vi "左相机穿管检测CCD1.vi"(8 "error in (no error)":errorcluster caption="错误输入（无错误）", 11 "名称或相对路径":string="Template Program") -> (0 "error in (no error) 2":errorcluster caption="错误输入（无错误）")   [LabVIEW 2017]
uses:
  Picture/SaveButtom.ctl
  <vilib>/vision/Pattern Matching.llb/IMAQ Curve Parameters.ctl
  Global System.vi
  <vilib>/Utility/xml.llb/Write to XML File(string).vi
panel:
  in  "ROI BIG 获取":bool
  in  "获取图像":bool
  in  "ROI LINE 获取":bool
  in  "创建模板":bool
  in  "保存图像":bool
  out "添加的路径":path
  in  "刷新":bool
  in  "测试按钮":bool
  in  "保存按钮":bool
  in  "Main":enum32{"主参数", "模板匹配参数 ", "CCD1 ROI参数", "测试效果"}(tab)
  in  "CCD1基础参数":T1={"IsNorImage"=TRUE, "Exposure Values"=100289, "ImagePath"=path "C:/Users/hedongpo/Desktop/514-hdp/Alignment Assemble System/Test Picture/B/3.bmp"} caption="参数界面" {"Exposure Values" scale=0.0..200000.0}
  in  "CCD1参数":T4={"Rectangle"={"Left"=1952, "Top"=146, "Right"=370, "Bottom"=2690, "Rotation"=45.0}, "Angle (degrees) "=90.0, "long"=150.0, "abgek"=-90.0, "Color"=16711680, "left threshold"=0.0, "Rectangle right"={"Left"=1952, "Top"=1596, "Right"=570, "Bottom"=2690, "Rotation"=45.0}, "long right"=150.0, "abgek right"=90.0, "Color 2"=16711680, "right threshold"=0.0, "left"=0.0, "right"=0.0, "Settings (Big)"={"Extraction Mode"=0, "Edge Threshold"=17, "Edge Filter Size"=1, "Min Length"=36, "Row Search Step Size"=13, "Col Search Step Size"=13, "Max Endpoint Gap"=10, "Closed"=FALSE, "Subpixel"=TRUE}, "Clamp Settings (Big)"={"Angle "=10.0, "Edge Polarity"={"Start"=0, "End"=0}}, " Settings top"={"Extraction Mode"=0, "Edge Threshold"=18, "Edge Filter Size"=1, "Min Length"=36, "Row Search Step Size"=64, "Col Search Step Size"=64, "Max Endpoint Gap"=10, "Closed"=FALSE, "Subpixel"=TRUE}, "Clamp Settings top "={"Angle "=10.0, "Edge Polarity"={"Start"=0, "End"=0}}, "Sub-Pixel Accuracy "=TRUE, "Threshold Parameters"={"Level Type"=enum."Absolute Value", "Threshold Level"=127, "Hysteresis"=2}, "Process "=enum."Get First + Last Edge", "Threshold Parameters 2"={"Level Type"=enum."Absolute Value", "Threshold Level"=127, "Hysteresis"=2}} {"Clamp Settings top"."Edge Polarity"."Start" items=["Any", "Rising", "Falling"]; "Clamp Settings top"."Edge Polarity"."End" items=["Any", "Rising", "Falling"]; "Settings top"."Extraction Mode" items=["Normal", "Uniform Regions"]; "Settings top"."Edge Filter Size" items=["Fine", "Normal", "Contour Tracing"]; "Settings top"."Max Endpoint Gap" min=0; "Settings top"."Col Search Step Size" min=1 max=255 step=1; "Settings top"."Row Search Step Size" min=1 max=255 step=1; "Settings top"."Min Length" min=0; "Settings top"."Edge Threshold" min=1 max=350 step=1; "Clamp Settings (Big)"."Edge Polarity"."Start" items=["Any", "Rising", "Falling"]; "Clamp Settings (Big)"."Edge Polarity"."End" items=["Any", "Rising", "Falling"]; "Settings (Big)"."Extraction Mode" items=["Normal", "Uniform Regions"]; "Settings (Big)"."Edge Filter Size" items=["Fine", "Normal", "Contour Tracing"]; "Settings (Big)"."Max Endpoint Gap" min=0; "Settings (Big)"."Col Search Step Size" min=1 max=255 step=1; "Settings (Big)"."Row Search Step Size" min=1 max=255 step=1; "Settings (Big)"."Min Length" min=0; "Settings (Big)"."Edge Threshold" min=1 max=350 step=1; "Rectangle right"."Rotation" format="%.2f"; "Rectangle right"."Left" scale=0.0..1024.0; "Rectangle right"."Right" scale=0.0..1024.0; "Rectangle"."Rotation" format="%.2f"; "Rectangle"."Left" scale=0.0..1024.0; "Rectangle"."Right" scale=0.0..1024.0}
  in  "CCD1 ROI参数":T6={"Rectangle big CCD1"={"Left"=1952, "Top"=1596, "Right"=570, "Bottom"=2690, "Rotation"=45.0}, "Rectangle top CCD1 "={"Left"=1952, "Top"=1596, "Right"=570, "Bottom"=2690, "Rotation"=45.0}, "Line"={"Start X"=0, "Start Y"=0, "End X"=0, "End Y"=0}, "left line "=846.0, "right line"=1152.0} {"Line"."Start X" scale=0.0..1024.0; "Line"."End X" scale=0.0..1024.0; "Rectangle top CCD1"."Rotation" format="%.2f"; "Rectangle top CCD1"."Left" scale=0.0..1024.0; "Rectangle top CCD1"."Right" scale=0.0..1024.0; "Rectangle big CCD1"."Rotation" format="%.2f"; "Rectangle big CCD1"."Left" scale=0.0..1024.0; "Rectangle big CCD1"."Right" scale=0.0..1024.0}
  out "原始图像":T7(plugin-control)
  out "路径输出":path
  in  "Vision Paramter Save Buttom":T8
  out "system time":string
  in  "取消按钮":bool
  # "箭头指示参数"
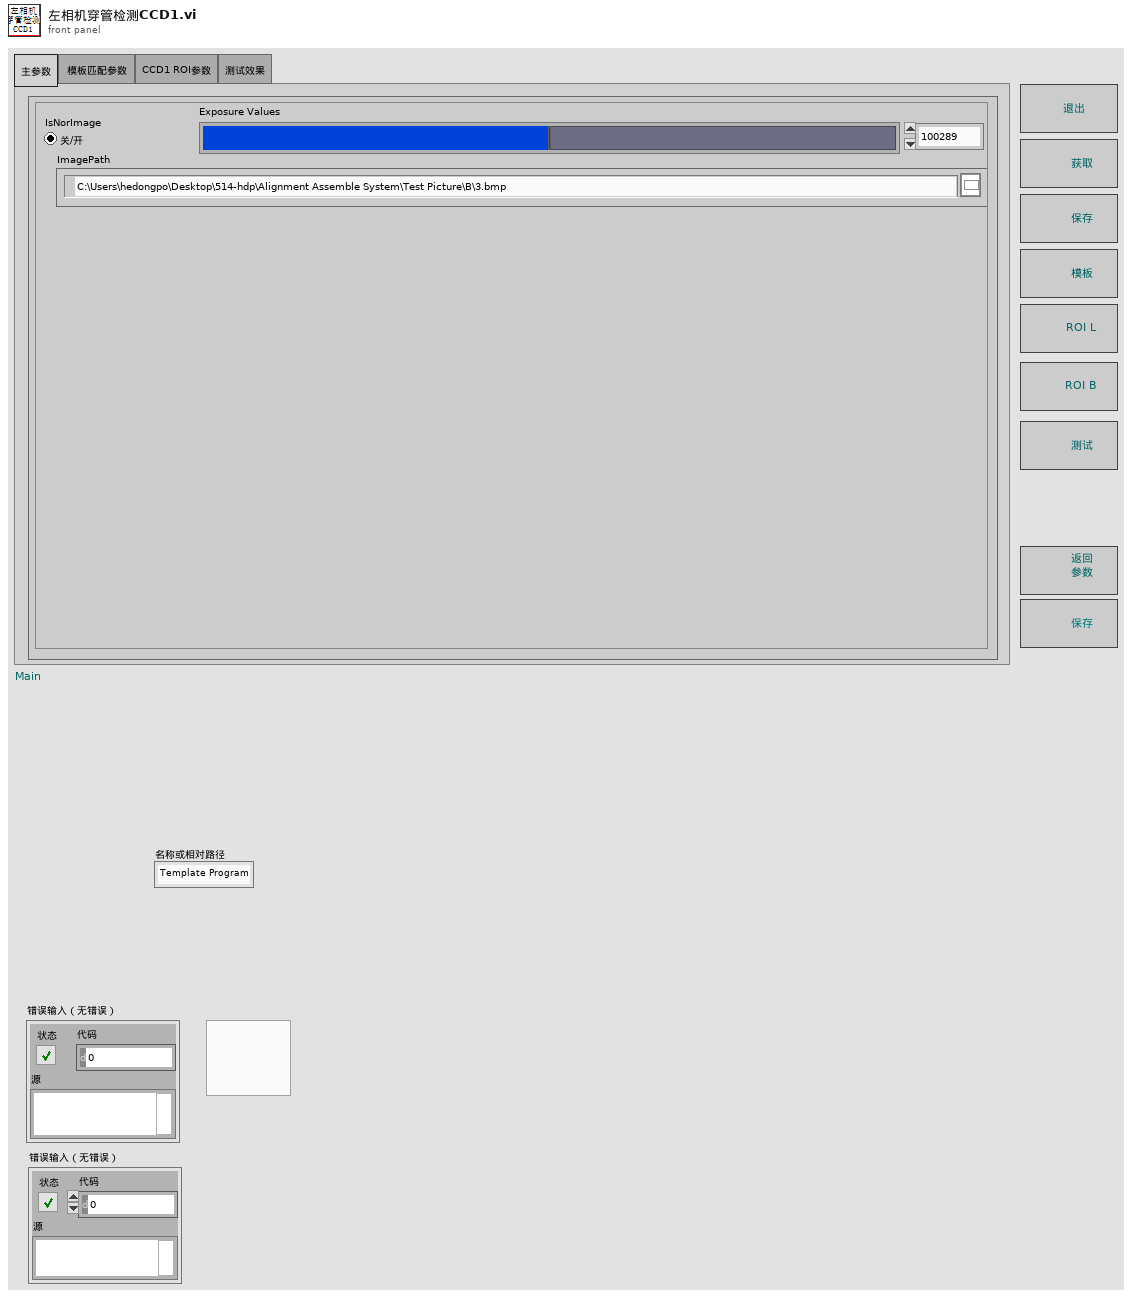
[diagram p1: front panel]
types:
  T1 = cluster{"IsNorImage":bool, "Exposure Values":u32, "ImagePath":path}
  T2 = typedef "IMAQ Rectangle" = cluster{"Left":i32, "Top":i32, "Right":i32, "Bottom":i32, "Rotation":dbl}
  T3 = typedef "IMAQ Curve Parameters.ctl" = cluster{"Extraction Mode":u32, "Edge Threshold":i32, "Edge Filter Size":u32, "Min Length":i32, "Row Search Step Size":i32, "Col Search Step Size":i32, "Max Endpoint Gap":i32, "Closed":bool, "Subpixel":bool}
  T4 = cluster{"Rectangle":T2, "Angle (degrees) ":sgl, "long":sgl, "abgek":dbl, "Color":u32, "left threshold":dbl, "Rectangle right":T2, "long right":sgl, "abgek right":dbl, "Color 2":u32, "right threshold":dbl, "left":dbl, "right":dbl, "Settings (Big)":T3, "Clamp Settings (Big)":cluster{"Angle ":dbl, "Edge Polarity":cluster{"Start":u32, "End":u32}}, " Settings top":T3, "Clamp Settings top ":cluster{"Angle ":dbl, "Edge Polarity":cluster{"Start":u32, "End":u32}}, "Sub-Pixel Accuracy ":bool, "Threshold Parameters":cluster{"Level Type":enum32{"Absolute Value", "Relative value"}, "Threshold Level":i32, "Hysteresis":i32}, "Process ":enum16{"Get First Edge", "Get First + Last Edge", "Get All Edges"}, "Threshold Parameters 2":cluster{"Level Type":enum32{"Absolute Value", "Relative value"}, "Threshold Level":i32, "Hysteresis":i32}}
  T5 = typedef "IMAQ Line" = cluster{"Start X":i32, "Start Y":i32, "End X":i32, "End Y":i32}
  T6 = cluster{"Rectangle big CCD1":T2, "Rectangle top CCD1 ":T2, "Line":T5, "left line ":dbl, "right line":dbl}
  T7 = typedef "IMAQ Image.ctl" = refnum<image>
  T8 = typedef "SaveButtom.ctl" = bool
  T9 = cluster{"index":i32, "this vi":refnum<vi>, "error out":errorcluster}
  T10 = cluster{"master data":string, "priority":u16, "secondary data":string[]}
  T11 = cluster{"case name":string[], "queue array":refnum<queue>[]}
  T12 = typedef "IMAQdx.ctl" = refnum<k21>
  T13 = cluster{"Global Rectangle":i32[], "Contours":cluster{"Contour Type":u32, "ROI Type":u32, "Points":i32[]}[]}
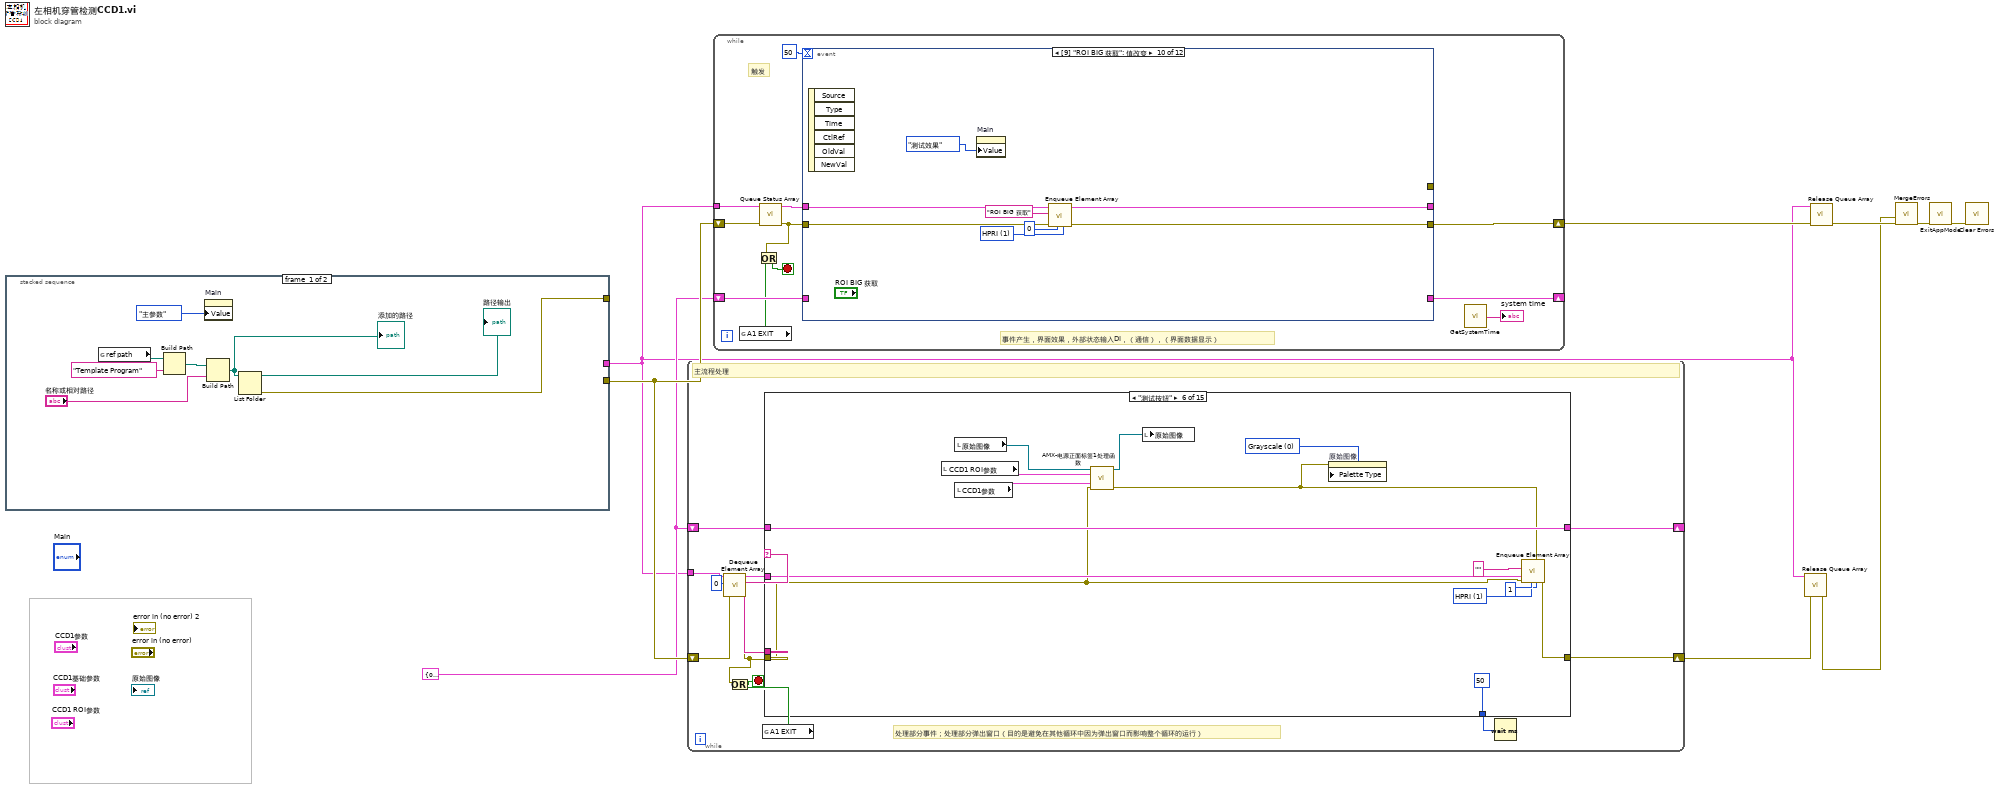
[diagram p0: block diagram]
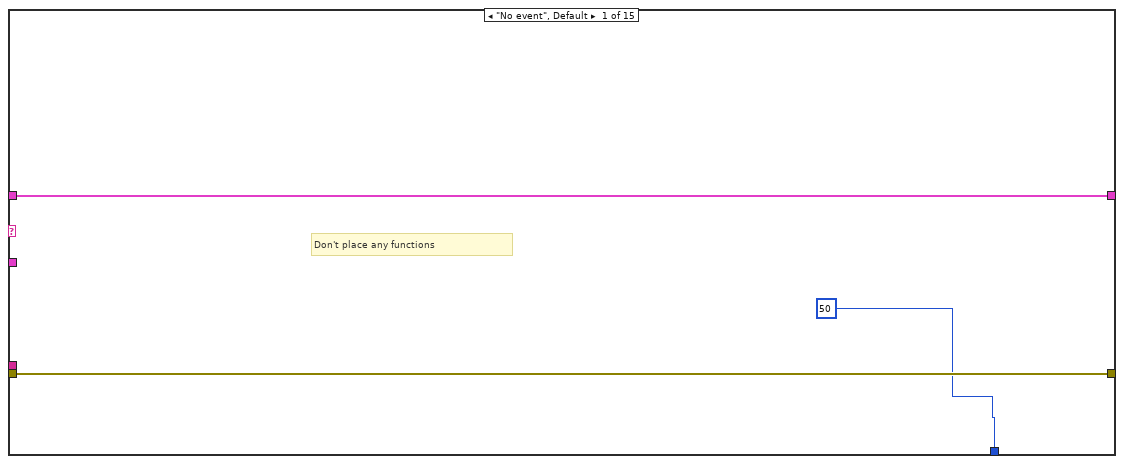
[diagram p2: hidden frame]
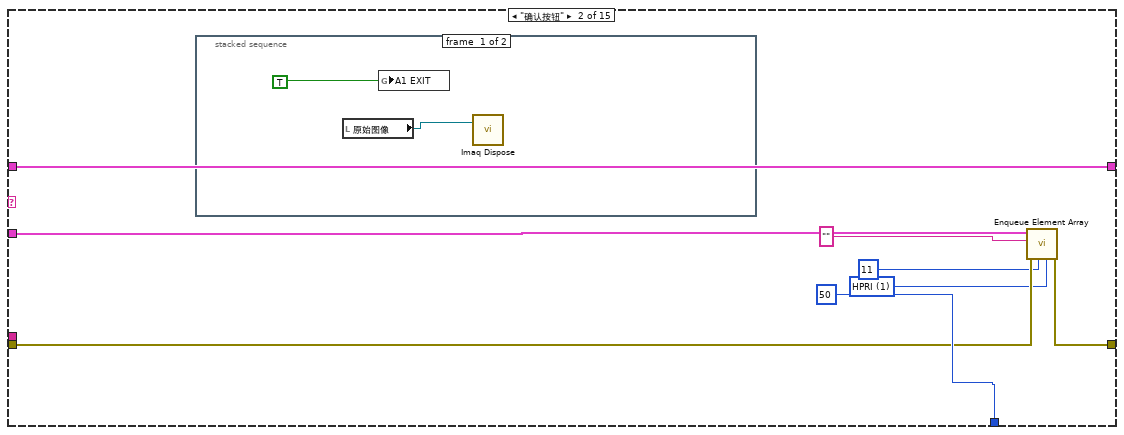
[diagram p3: hidden frame]
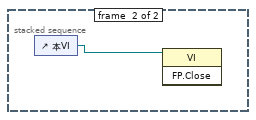
[diagram p4: hidden frame]
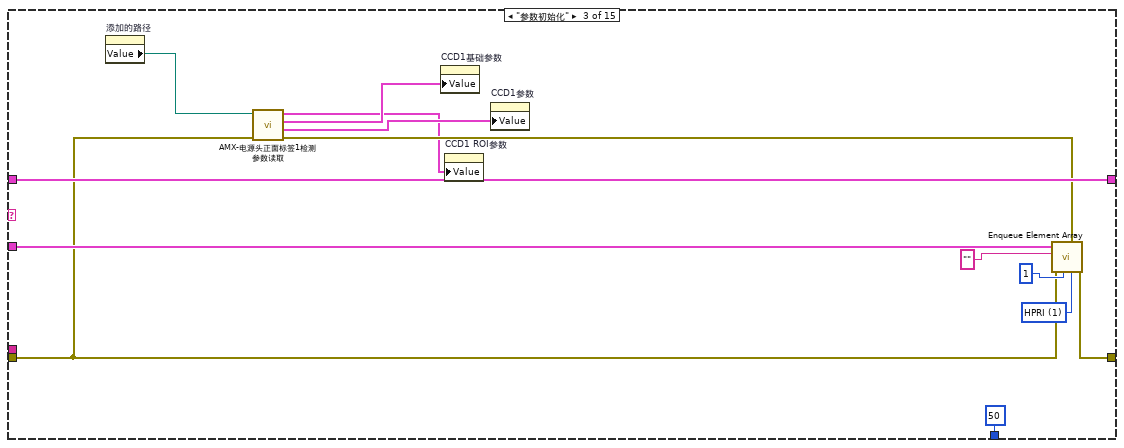
[diagram p5: hidden frame]
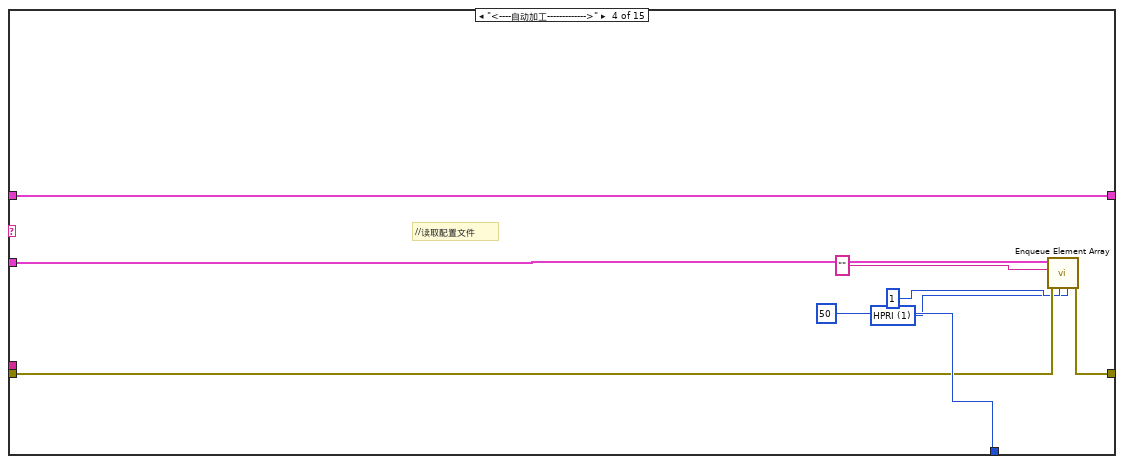
[diagram p6: hidden frame]
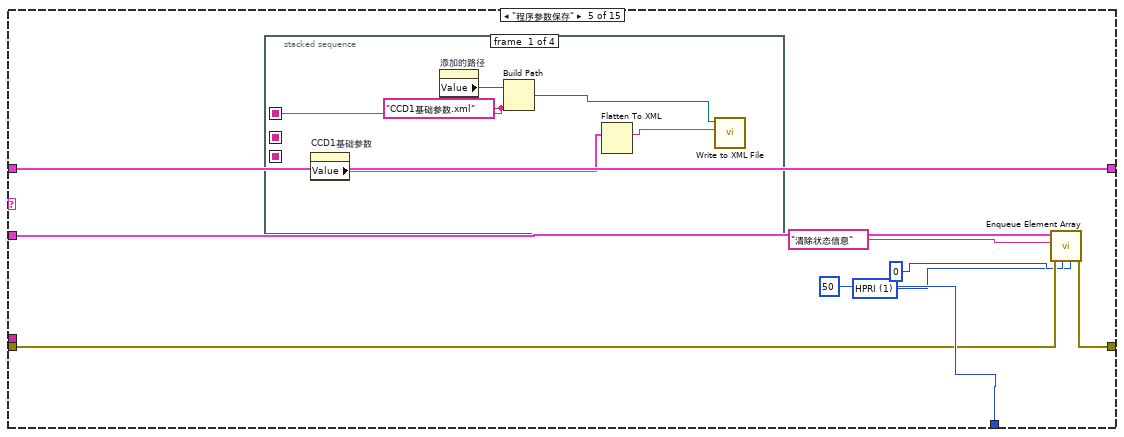
[diagram p7: hidden frame]
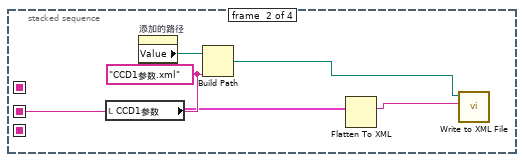
[diagram p8: hidden frame]
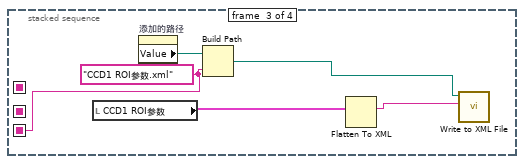
[diagram p9: hidden frame]
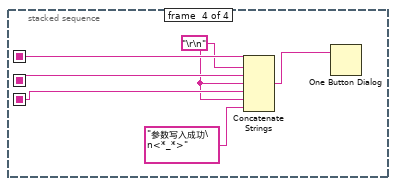
[diagram p10: hidden frame]
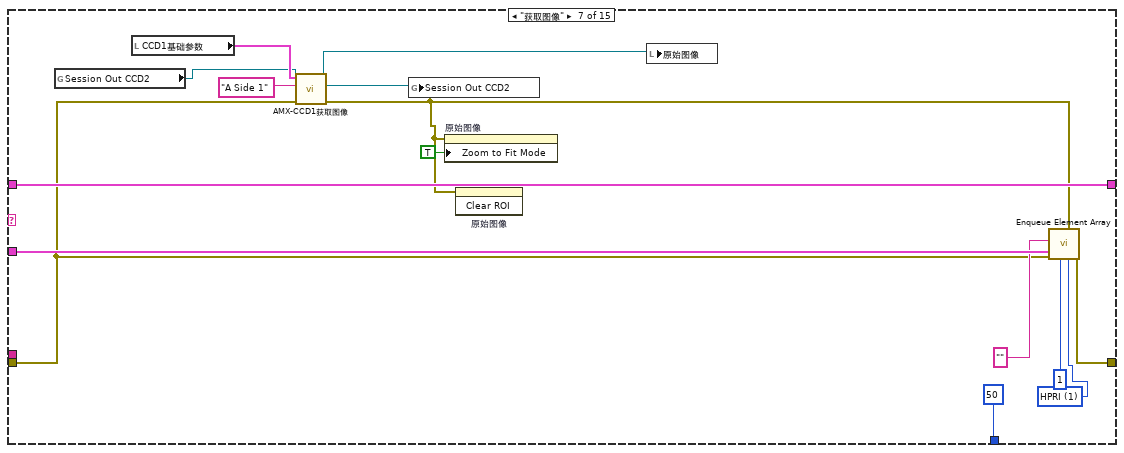
[diagram p11: hidden frame]
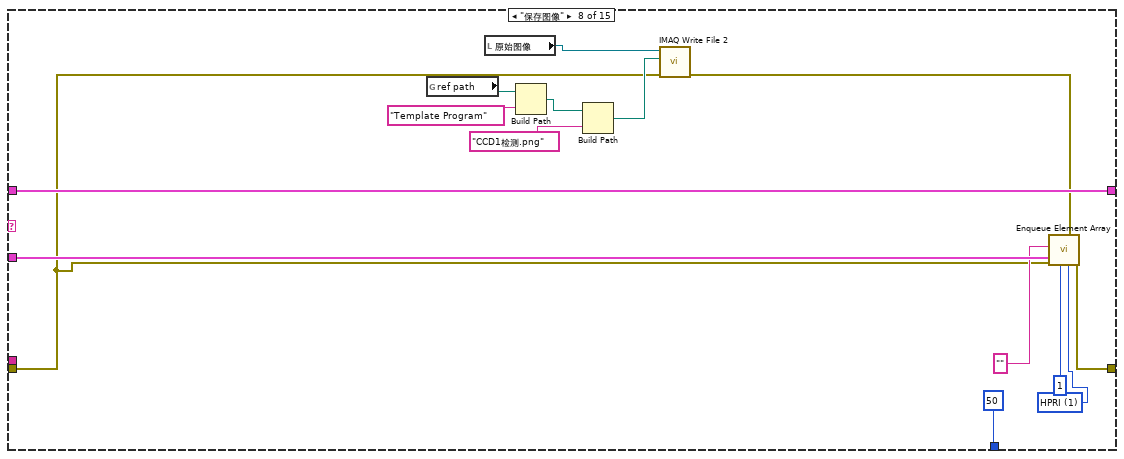
[diagram p12: hidden frame]
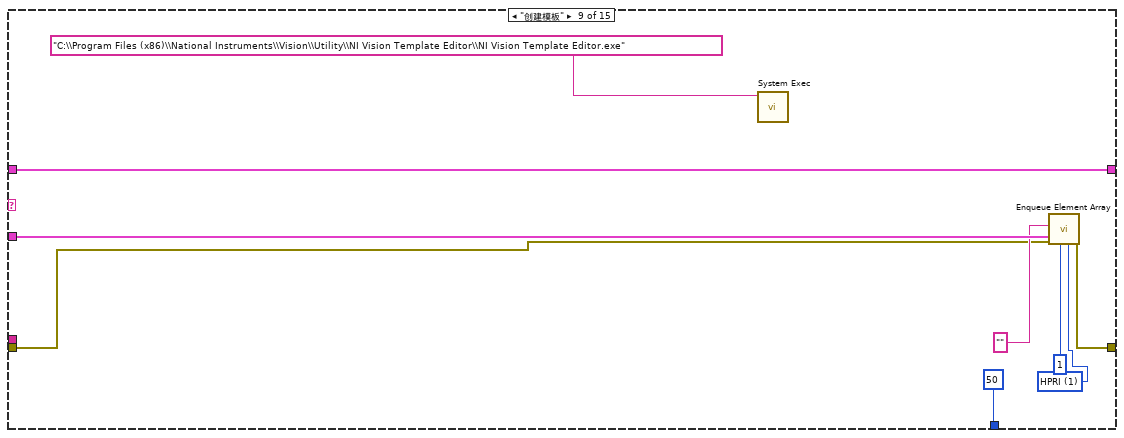
[diagram p13: hidden frame]
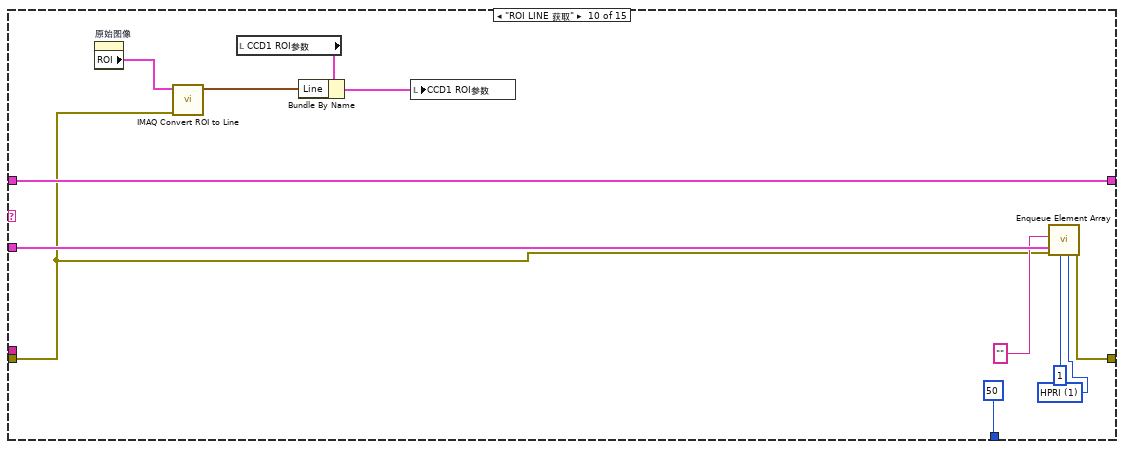
[diagram p14: hidden frame]
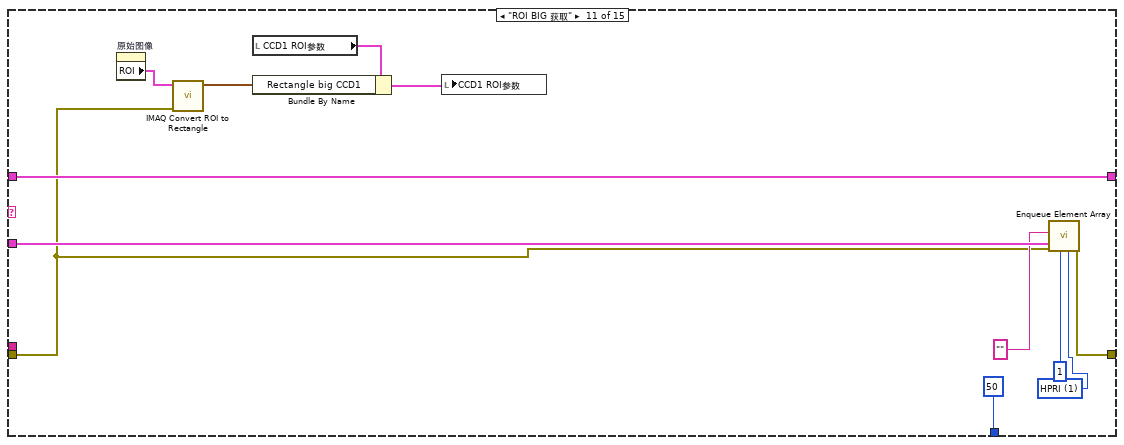
[diagram p15: hidden frame]
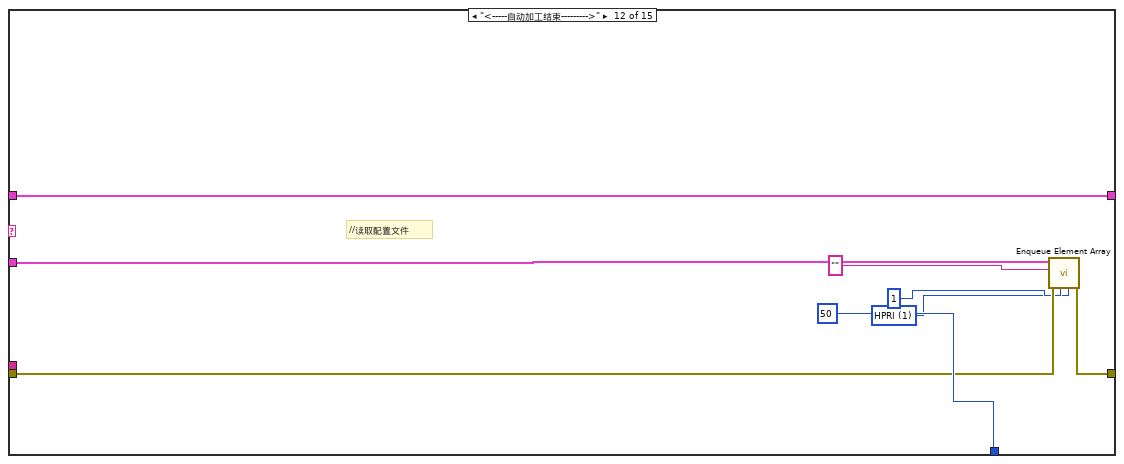
[diagram p16: hidden frame]
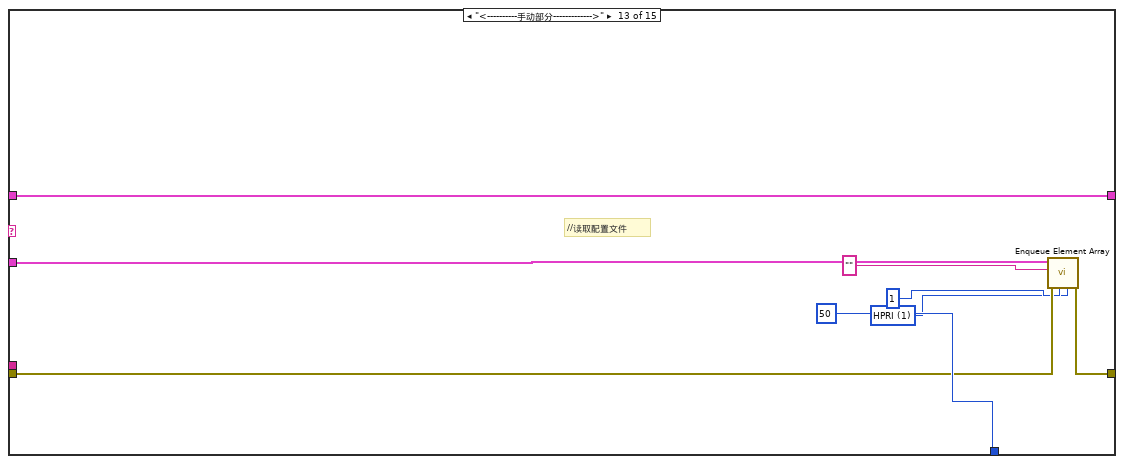
[diagram p17: hidden frame]
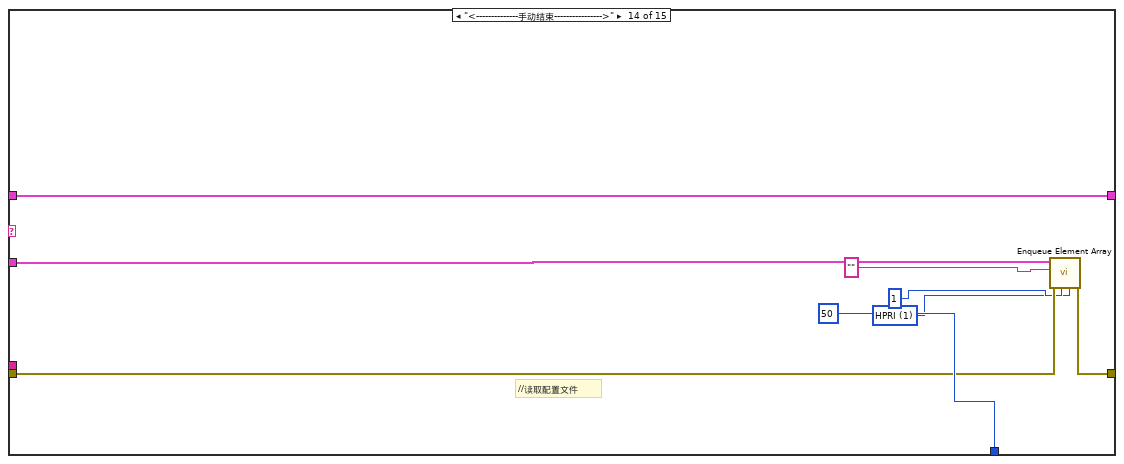
[diagram p18: hidden frame]
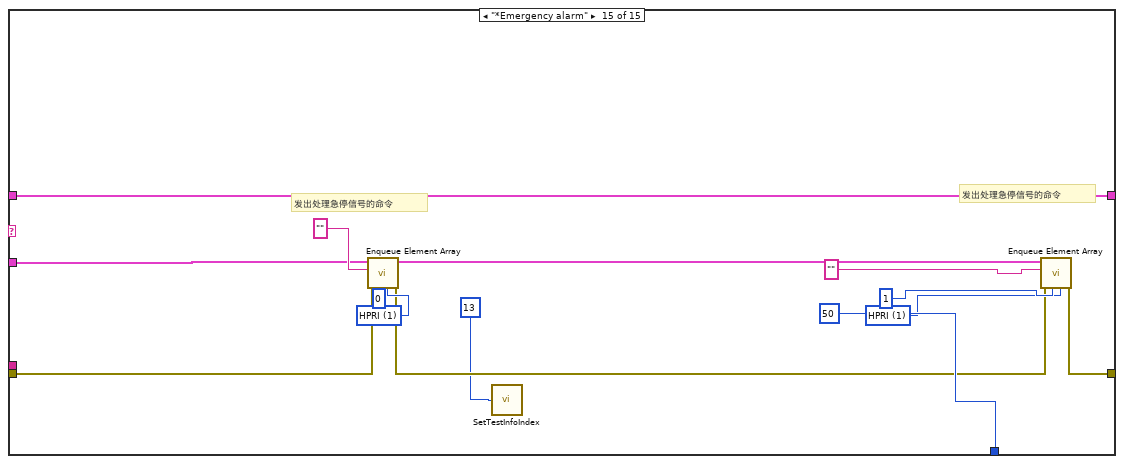
[diagram p19: hidden frame]
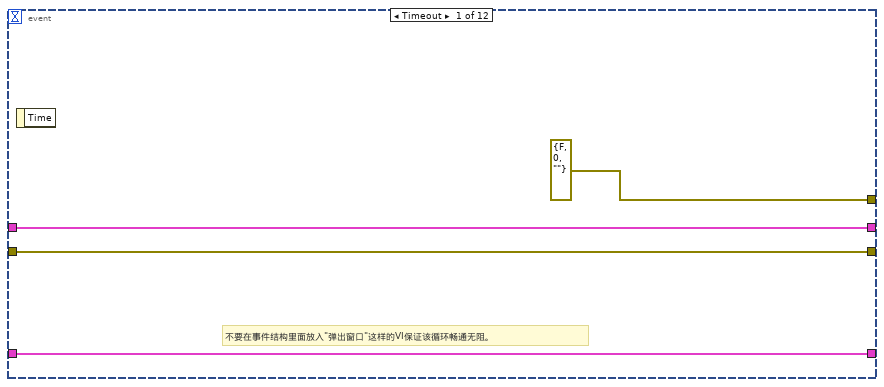
[diagram p20: hidden frame]
diagram:
  w4 = T9 {"index"=0, "this vi"=refnum, "error out"={"status"=FALSE, "code"=0, "source"=""}} ("parameter buffer")
  n1 = stacked-sequence {
    tunnel: [w15 _] -> _
    tunnel: [_ w19] -> w5
    tunnel: [_ w18] -> w1
    frame #0 {
      n2 = global read "Global System.vi" "ref path"() -> (w13:path)
      n3 = Build Path(base path=w13, name or relative path="Template Program" ("名称或相对路径")) -> (appended path=w11:path)
      n4 = property on="Main" class="TabCtl (严格)"("Value"=enum32{"主参数", "模板匹配参数 ", "CCD1 ROI参数", "测试效果"}."主参数" ("Main")) -> ()  [unwired: 2 in, 2 out]
      n5 = Build Path(base path=w11, name or relative path="名称或相对路径") -> (appended path=w17:path)
      "添加的路径" <- w17
      n6 = List Folder(path=w17) -> (path out=→"路径输出":path, error out=w15:errorcluster)  [unwired: 3 in, 2 out]
    }
    frame #1 {
      w27 = string[] ["comm queue1", "data queue 11", "data queue 12", "data queue 13", "data queue 14"]  # queue name
      w28 = 4  # queue num
      w29 = T10 {"master data"="", "priority"=0, "secondary data"=[]}  # element data type
      n7 = call "Obtain Queue Array.vi"("queue name"=w27, "element data type"=w29, "queue num"=w28) -> ("error out"=w23:errorcluster, "queue out"=w24:T11)  [unwired: 2 in, 1 out]
      n8 = call "Enqueue Element Array.vi"("queue index"=0, "error in"=w23, "master data"="参数初始化", "queue in"=w24) -> ("error out"=w22:errorcluster, "queue out"=w21:T11)  [unwired: 6 in]
      n9 = disable-structure shown="启用" {
        disable-tunnel: w22 -> [w35 w36]
        disable-tunnel: w21 -> [w34 w37]
        disable-tunnel: "Loading Variable" ("master data") -> [w33 _]
        disable-tunnel: [w31 w36] -> w19
        disable-tunnel: [w30 w37] -> w18
        frame Disabled {
          n10 = call "Enqueue Element Array.vi"("queue index"=12, "error in"=w35, "master data"=w33, "queue in"=w34) -> ("error out"=w31:errorcluster, "queue out"=w30:T11)  [unwired: 6 in]
        }
        frame Enabled {
        }
      }
    }
  }
  n11 = while {
    shift-right: [w50] -> w3
    shift-left: w5 -> [w41]
    shift-right: [w47] -> _
    shift-left: w4 -> [w48]
    tunnel: w1 -> [w43]
    stop <- w38 stop-if-true
    # "处理部分事件；处理部分弹出窗口（目的是避免在其他循环中因为弹出窗口而影响整个循环的运行）"
    # "主流程处理"
    n12 = call "Dequeue Element Array.vi"("queue in"=w43, "queue index"=0, "error in"=w41) -> ("queue out"=w46:T11, "master data"=w45:string, "secondary data"=w44:string[], "error out"=w40:errorcluster)  [unwired: 2 in, 1 out]
    n13 = global read "Global System.vi" "A1 EXIT"() -> (w39:bool)
    n14 = Or(x=w40, y=w39) -> (x .or. y?=w38:bool)
    n15 = case shown="\"测试按钮\"" w45 {
      tunnel: w46 -> [_ w60 w76 w84 w86 w127 w142 w157 w166 w178 w190 w198 w206 w214 w220]
      tunnel: w40 -> [w52 w56 w69 w80 w90 w121 w133 w144 w160 w171 w183 w194 w202 w210 w217]
      tunnel: [w52 w59 w75 w83 w92 w126 w141 w156 w165 w177 w189 w197 w205 w213 w228] -> w50
      tunnel: [50 50 50 50 50 50 50 50 50 50 50 50 50 50 50] -> w49
      tunnel: w48 -> [w53 w57 w71 w81 w87 w122 w137 w152 w161 w173 w185 w195 w203 w211 w226]
      tunnel: [w53 w57 w71 w81 w87 w122 w137 w152 w161 w173 w185 w195 w203 w211 w226] -> w47
      tunnel: w44 -> [_ _ _ _ _ _ _ _ _ _ _ _ _ _ _]
      frame "No event", Default {
        # "Don't place any functions"
      }
      frame "确认按钮" {
        w54 = u16 1 items=["HPRI"=1, "LPRI"=0] ("priority")
        n16 = stacked-sequence {
          frame #0 {
            n17 = local read "原始图像"() -> (w62:T7)
            n18 = global write "Global System.vi" "A1 EXIT"(TRUE ("EXIT")) -> ()
            n19 = call "Imaq Dispose"("Image"=w62) -> ()  [unwired: 5 in, 1 out]
          }
          frame #1 {
            n20 = control-ref of="本VI"() -> (w64:refnum<vi>)
            n21 = invoke class="VI" method="FP.Close"(reference=w64) -> ()  [unwired: 2 in, 3 out]
          }
        }
        n22 = call "Enqueue Element Array.vi"("priority"=w54, "queue index"=11, "error in"=w56, "master data"="" ("Element 1"), "queue in"=w60) -> ("error out"=w59:errorcluster)  [unwired: 5 in, 1 out]
      }
      frame "参数初始化" {
        w72 = u16 1 items=["HPRI"=1, "LPRI"=0] ("priority")
        n23 = property on="添加的路径" class="Path"() -> ("Value"=w70:path)  [unwired: 2 in, 2 out]
        n24 = call "AMX-电源头正面标签1检测参数读取.vi"("error in (no error)"=w69, "基路径"=w70) -> ("error out"=w68:errorcluster, "CCD1参数"=w66:T4, "CCD1基础参数"=w67:T1, "CCD1 ROI参数"=w65:T6)  [unwired: 5 in]
        n25 = property on="CCD1基础参数" class="Clust (严格)"("Value"=w67) -> ()  [unwired: 2 in, 2 out]
        n26 = property on="CCD1 ROI参数" class="Clust (严格)"("Value"=w65) -> ()  [unwired: 2 in, 2 out]
        n27 = property on="CCD1参数" class="Clust (严格)"("Value"=w66) -> ()  [unwired: 2 in, 2 out]
        n28 = call "Enqueue Element Array.vi"("priority"=w72, "device error in"=w68, "queue index"=1, "error in"=w69, "master data"="" ("Element 1"), "queue in"=w76) -> ("error out"=w75:errorcluster)  [unwired: 4 in, 1 out]
      }
      frame "<----自动加工------------->" {
        w78 = u16 1 items=["HPRI"=1, "LPRI"=0] ("priority")
        # "//读取配置文件"
        n29 = call "Enqueue Element Array.vi"("priority"=w78, "queue index"=1, "error in"=w80, "master data"="" ("Element 1"), "queue in"=w84) -> ("error out"=w83:errorcluster)  [unwired: 5 in, 1 out]
      }
      frame "程序参数保存" {
        w88 = u16 1 items=["HPRI"=1, "LPRI"=0] ("priority")
        n30 = stacked-sequence {
          seq-local: [w94 _ _ _] -> [_ _ _ w114]
          seq-local: [_ w100 _ _] -> [_ _ _ w112]
          seq-local: [_ _ w104 _] -> [_ _ _ w110]
          frame #0 {
            w94 = "CCD1基础参数.xml" ("名称或相对路径")
            n31 = property on="CCD1基础参数" class="Clust (严格)"() -> ("Value"=w97:T1)  [unwired: 2 in, 2 out]
            n32 = property on="添加的路径" class="Path"() -> ("Value"=w98:path)  [unwired: 2 in, 2 out]
            n33 = Build Path(base path=w98, name or relative path=w94) -> (appended path=w95:path)
            n34 = Flatten To XML(anything=w97) -> (xml string=w96:string)
            n35 = call-poly <vilib>:"Write to XML File.vi"("XML Input"=w96, "XML File Path"=w95) -> ()  [unwired: 7 in, 3 out]
          }
          frame #1 {
            w100 = "CCD1参数.xml" ("名称或相对路径")
            n36 = local read "CCD1参数"() -> (w99:T4)
            n37 = property on="添加的路径" class="Path"() -> ("Value"=w103:path)  [unwired: 2 in, 2 out]
            n38 = Build Path(base path=w103, name or relative path=w100) -> (appended path=w101:path)
            n39 = Flatten To XML(anything=w99) -> (xml string=w102:string)
            n40 = call-poly <vilib>:"Write to XML File.vi"("XML Input"=w102, "XML File Path"=w101) -> ()  [unwired: 7 in, 3 out]
          }
          frame #2 {
            w104 = "CCD1 ROI参数.xml" ("名称或相对路径")
            n41 = local read "CCD1 ROI参数"() -> (w105:T6)
            n42 = property on="添加的路径" class="Path"() -> ("Value"=w108:path)  [unwired: 2 in, 2 out]
            n43 = Build Path(base path=w108, name or relative path=w104) -> (appended path=w106:path)
            n44 = Flatten To XML(anything=w105) -> (xml string=w107:string)
            n45 = call-poly <vilib>:"Write to XML File.vi"("XML Input"=w107, "XML File Path"=w106) -> ()  [unwired: 7 in, 3 out]
          }
          frame #3 {
            w109 = "\r\n"
            n46 = Concatenate Strings(w114, w109, w112, w109, w110, w109, "参数写入成功\n<*_*>" ("消息")) -> (w113:string)
            n47 = One Button Dialog(message=w113) -> ()  [unwired: 1 in, 1 out]
          }
        }
        n48 = call "Enqueue Element Array.vi"("priority"=w88, "queue index"=0, "error in"=w90, "master data"="清除状态信息" ("Element 1"), "queue in"=w86) -> ("error out"=w92:errorcluster)  [unwired: 5 in, 1 out]
      }
      frame "测试按钮" {
        w119 = u32 0 items=["Grayscale", "Binary", "Gradient", "Rainbow", "Temperature", "User Defined", "Binary 16 Bit", "Gradient 16 Bit", "Rainbow 16 Bit", "Temperature 16 Bit", "User Defined 16 Bit"] ("Palette:Palette Type")
        w123 = u16 1 items=["HPRI"=1, "LPRI"=0] ("priority")
        n49 = local read "CCD1 ROI参数"() -> (w115:T6)
        n50 = local read "原始图像"() -> (w120:T7)
        n51 = local read "CCD1参数"() -> (w116:T4)
        n52 = call "AMX-电源正面标签1处理函数.vi"("Image in"=w120, "ROI参数"=w115, "CCD1参数"=w116, "error in (no error)"=w121) -> ("Image out"=w117:T7, "error out"=w118:errorcluster)  [unwired: 7 in, 3 out]
        n53 = local write "原始图像"(w117) -> ()
        n54 = property on="原始图像" class="ImageControl"(error in=w118, "Palette Type"=w119) -> ()  [unwired: 1 in, 2 out]
        n55 = call "Enqueue Element Array.vi"("priority"=w123, "device error in"=w118, "queue index"=1, "error in"=w121, "master data"="" ("Element 1"), "queue in"=w127) -> ("error out"=w126:errorcluster)  [unwired: 4 in, 1 out]
      }
      frame "获取图像" {
        w138 = u16 1 items=["HPRI"=1, "LPRI"=0] ("priority")
        n56 = global read "Global System.vi" "Session Out CCD2"() -> (w130:T12)
        n57 = local read "CCD1基础参数"() -> (w135:T1)
        n58 = call "AMX-CCD1获取图像.vi"("Session Out CCD2"=w130, "error in (no error)"=w133, "Image Name"="A Side 1", "ParamsUI"=w135) -> ("error out"=w131:errorcluster, "Session Out"=w129:T12, "Image out"=w134:T7)  [unwired: 4 in, 1 out]
        n59 = global write "Global System.vi" "Session Out CCD2"(w129) -> ()
        n60 = property on="原始图像" class="ImageControl"(error in=w131, "Zoom to Fit Mode"=TRUE) -> ()  [unwired: 1 in, 2 out]
        n61 = invoke on="原始图像" class="ImageControl" method="Clear ROI"(error in=w131) -> ()  [unwired: 2 in, 3 out]
        n62 = local write "原始图像"(w134) -> ()
        n63 = call "Enqueue Element Array.vi"("priority"=w138, "device error in"=w131, "queue index"=1, "error in"=w133, "master data"="" ("Element 1"), "queue in"=w142) -> ("error out"=w141:errorcluster)  [unwired: 4 in, 1 out]
      }
      frame "保存图像" {
        w153 = u16 1 items=["HPRI"=1, "LPRI"=0] ("priority")
        n64 = global read "Global System.vi" "ref path"() -> (w151:path)
        n65 = local read "原始图像"() -> (w145:T7)
        n66 = Build Path(base path=w151, name or relative path="Template Program" ("名称或相对路径")) -> (appended path=w149:path)
        n67 = Build Path(base path=w149, name or relative path="CCD1检测.png" ("名称或相对路径")) -> (appended path=w147:path)
        n68 = call-poly "IMAQ Write File 2"("error in (no error)"=w144, "File Path"=w147, "Image"=w145) -> ("error out"=w146:errorcluster)  [unwired: 7 in, 1 out]
        n69 = call "Enqueue Element Array.vi"("priority"=w153, "device error in"=w146, "queue index"=1, "error in"=w144, "master data"="" ("Element 1"), "queue in"=w157) -> ("error out"=w156:errorcluster)  [unwired: 4 in, 1 out]
      }
      frame "创建模板" {
        w162 = u16 1 items=["HPRI"=1, "LPRI"=0] ("priority")
        n70 = call <vilib>:"System Exec.vi"("command line"="C:\\Program Files (x86)\\National Instruments\\Vision\\Utility\\NI Vision Template Editor\\NI Vision Template Editor.exe") -> ()  [unwired: 7 in, 4 out]
        n71 = call "Enqueue Element Array.vi"("priority"=w162, "queue index"=1, "error in"=w160, "master data"="" ("Element 1"), "queue in"=w166) -> ("error out"=w165:errorcluster)  [unwired: 5 in, 1 out]
      }
      frame "ROI LINE 获取" {
        w174 = u16 1 items=["HPRI"=1, "LPRI"=0] ("priority")
        n72 = property on="原始图像" class="ImageControl"() -> ("ROI"=w172:T13)  [unwired: 2 in, 2 out]
        n73 = call "IMAQ Convert ROI to Line"("error in (no error)"=w171, "ROI Descriptor"=w172) -> ("Line"=w170:T5)  [unwired: 7 in, 1 out]
        n74 = local read "CCD1 ROI参数"() -> (w169:T6)
        n75 = Bundle By Name(cluster=w169, "Line"=w170) -> (w168:T6)
        n76 = local write "CCD1 ROI参数"(w168) -> ()
        n77 = call "Enqueue Element Array.vi"("priority"=w174, "queue index"=1, "error in"=w171, "master data"="" ("Element 1"), "queue in"=w178) -> ("error out"=w177:errorcluster)  [unwired: 5 in, 1 out]
      }
      frame "ROI BIG 获取" {
        w186 = u16 1 items=["HPRI"=1, "LPRI"=0] ("priority")
        n78 = property on="原始图像" class="ImageControl"() -> ("ROI"=w184:T13)  [unwired: 2 in, 2 out]
        n79 = call "IMAQ Convert ROI to Rectangle"("error in (no error)"=w183, "ROI Descriptor"=w184) -> ("Rectangle"=w182:T2)  [unwired: 7 in, 1 out]
        n80 = local read "CCD1 ROI参数"() -> (w181:T6)
        n81 = Bundle By Name(cluster=w181, "Rectangle big CCD1"=w182) -> (w180:T6)
        n82 = local write "CCD1 ROI参数"(w180) -> ()
        n83 = call "Enqueue Element Array.vi"("priority"=w186, "queue index"=1, "error in"=w183, "master data"="" ("Element 1"), "queue in"=w190) -> ("error out"=w189:errorcluster)  [unwired: 5 in, 1 out]
      }
      frame "<-----自动加工结束--------->" {
        w192 = u16 1 items=["HPRI"=1, "LPRI"=0] ("priority")
        # "//读取配置文件"
        n84 = call "Enqueue Element Array.vi"("priority"=w192, "queue index"=1, "error in"=w194, "master data"="" ("Element 1"), "queue in"=w198) -> ("error out"=w197:errorcluster)  [unwired: 5 in, 1 out]
      }
      frame "<----------手动部分------------->" {
        w200 = u16 1 items=["HPRI"=1, "LPRI"=0] ("priority")
        # "//读取配置文件"
        n85 = call "Enqueue Element Array.vi"("priority"=w200, "queue index"=1, "error in"=w202, "master data"="" ("Element 1"), "queue in"=w206) -> ("error out"=w205:errorcluster)  [unwired: 5 in, 1 out]
      }
      frame "<--------------手动结束---------------->" {
        w208 = u16 1 items=["HPRI"=1, "LPRI"=0] ("priority")
        # "//读取配置文件"
        n86 = call "Enqueue Element Array.vi"("priority"=w208, "queue index"=1, "error in"=w210, "master data"="" ("Element 1"), "queue in"=w214) -> ("error out"=w213:errorcluster)  [unwired: 5 in, 1 out]
      }
      frame "*Emergency alarm" {
        w223 = u16 1 items=["HPRI"=1, "LPRI"=0] ("priority")
        w224 = u16 1 items=["HPRI"=1, "LPRI"=0] ("priority")
        # "发出处理急停信号的命令"
        # "发出处理急停信号的命令"
        n87 = call "Enqueue Element Array.vi"("priority"=w223, "queue index"=0, "error in"=w217, "master data"="" ("Element 1"), "queue in"=w220) -> ("error out"=w218:errorcluster, "queue out"=w219:T11)  [unwired: 5 in]
        n88 = call "SetTestInfoIndex.vi"("test info index"=13) -> ()
        n89 = call "Enqueue Element Array.vi"("priority"=w224, "queue index"=1, "error in"=w218, "master data"="" ("Element 1"), "queue in"=w219) -> ("error out"=w228:errorcluster)  [unwired: 5 in, 1 out]
      }
    }
    n90 = Wait (ms)(milliseconds to wait=w49) -> ()  [unwired: 1 out]
  }
  n91 = while {
    shift-right: [w233] -> w6
    shift-left: w5 -> [w237]
    shift-right: [w235] -> _
    shift-left: w4 -> [w236]
    tunnel: w1 -> [w239]
    stop <- w230 stop-if-true
    # "触发"
    # "事件产生，界面效果，外部状态输入DI，（通信），（界面数据显示）"
    n92 = global read "Global System.vi" "A1 EXIT"() -> (w231:bool)
    n93 = call "Queue Status Array.vi"("error in (no error)"=w237, "queue in"=w239) -> ("error out"=w232:errorcluster, "queue out"=w234:T11)  [unwired: 4 in]
    n94 = Or(x=w232, y=w231) -> (x .or. y?=w230:bool)
    n95 = event shown="[9] \"ROI BIG 获取\": 值改变" {
      selector: _ -> [_ _ _ _ _ _ _ _ _ _ _ _]
      dyn-events: _ -> [_ _ _ _ _ _ _ _ _ _ _ _]
      timeout: 50 -> [_ _ _ _ _ _ _ _ _ _ _ _]
      tunnel: w236 -> [w244 w252 _ _ _ _ _ _ _ _ _ _]
      tunnel: [w244 w252 _ _ _ _ _ _ _ _ _ _] -> w235
      tunnel: [errorcluster {"status"=FALSE, "code"=0, "source"=""} ("error out") _ _ _ _ _ _ _ _ _ _ _] -> _
      tunnel: w234 -> [w242 w251 w257 w264 w271 w279 w286 w293 w301 w309 w317 w325]
      tunnel: w232 -> [w241 w250 w256 w263 w270 w278 w285 w292 w300 w308 w316 w324]
      tunnel: [w241 w249 w254 w261 w268 w276 w283 w290 w298 w306 w314 w322] -> w233
      tunnel: [w242 w248 w255 w262 w269 w277 w284 w291 w299 w307 w315 w323] -> _
      event Timeout {
        # "不要在事件结构里面放入\"弹出窗口\"这样的VI保证该循环畅通无阻。"
        n96 = event-data() -> ()  [unwired: 1 in, 1 out]
      }
      event Panel Close? {
        w246 = u16 1 items=["HPRI"=1, "LPRI"=0] ("priority")
        n97 = event-data() -> ()  [unwired: 1 in, 4 out]
        n98 = call "Enqueue Element Array.vi"("priority"=w246, "queue index"=0, "error in"=w250, "master data"="*Exit application", "queue in"=w251) -> ("error out"=w249:errorcluster, "queue out"=w248:T11)  [unwired: 5 in]
        n99 = event-data("Discard?"=TRUE) -> ()  [unwired: 1 in, 1 out]
      }
      event Value Change {
        w259 = u16 1 items=["HPRI"=1, "LPRI"=0] ("priority")
        n100 = event-data() -> ()  [unwired: 1 in, 6 out]
        n101 = call "Enqueue Element Array.vi"("priority"=w259, "queue index"=0, "error in"=w256, "master data"="Vision Paramter Save", "queue in"=w257) -> ("error out"=w254:errorcluster, "queue out"=w255:T11)  [unwired: 5 in]
      }
      event "取消按钮": Value Change {
        w266 = u16 1 items=["HPRI"=1, "LPRI"=0] ("priority")
        n102 = event-data() -> ()  [unwired: 1 in, 6 out]
        n103 = call "Enqueue Element Array.vi"("priority"=w266, "queue index"=0, "error in"=w263, "master data"="确认按钮", "queue in"=w264) -> ("error out"=w261:errorcluster, "queue out"=w262:T11)  [unwired: 5 in]
      }
      event "保存按钮": Value Change {
        w273 = u16 1 items=["HPRI"=1, "LPRI"=0] ("priority")
        n104 = event-data() -> ()  [unwired: 1 in, 6 out]
        n105 = call "Enqueue Element Array.vi"("priority"=w273, "queue index"=0, "error in"=w270, "master data"="程序参数保存", "queue in"=w271) -> ("error out"=w268:errorcluster, "queue out"=w269:T11)  [unwired: 5 in]
      }
      event "获取图像": Value Change {
        w281 = u16 1 items=["HPRI"=1, "LPRI"=0] ("priority")
        n106 = event-data() -> ()  [unwired: 1 in, 6 out]
        n107 = property on="Main" class="TabCtl (严格)"("Value"=enum32{"主参数", "模板匹配参数 ", "CCD1 ROI参数", "测试效果"}."测试效果" ("Main")) -> ()  [unwired: 2 in, 2 out]
        n108 = call "Enqueue Element Array.vi"("priority"=w281, "queue index"=0, "error in"=w278, "master data"="获取图像", "queue in"=w279) -> ("error out"=w276:errorcluster, "queue out"=w277:T11)  [unwired: 5 in]
      }
      event "保存图像": Value Change {
        w288 = u16 1 items=["HPRI"=1, "LPRI"=0] ("priority")
        n109 = event-data() -> ()  [unwired: 1 in, 6 out]
        n110 = call "Enqueue Element Array.vi"("priority"=w288, "queue index"=0, "error in"=w285, "master data"="保存图像", "queue in"=w286) -> ("error out"=w283:errorcluster, "queue out"=w284:T11)  [unwired: 5 in]
      }
      event "创建模板": Value Change {
        w295 = u16 1 items=["HPRI"=1, "LPRI"=0] ("priority")
        n111 = event-data() -> ()  [unwired: 1 in, 6 out]
        n112 = call "Enqueue Element Array.vi"("priority"=w295, "queue index"=0, "error in"=w292, "master data"="创建模板", "queue in"=w293) -> ("error out"=w290:errorcluster, "queue out"=w291:T11)  [unwired: 5 in]
      }
      event "ROI LINE 获取": Value Change {
        w303 = u16 1 items=["HPRI"=1, "LPRI"=0] ("priority")
        n113 = event-data() -> ()  [unwired: 1 in, 6 out]
        n114 = property on="Main" class="TabCtl (严格)"("Value"=enum32{"主参数", "模板匹配参数 ", "CCD1 ROI参数", "测试效果"}."测试效果" ("Main")) -> ()  [unwired: 2 in, 2 out]
        n115 = call "Enqueue Element Array.vi"("priority"=w303, "queue index"=0, "error in"=w300, "master data"="ROI LINE 获取", "queue in"=w301) -> ("error out"=w298:errorcluster, "queue out"=w299:T11)  [unwired: 5 in]
      }
      event "ROI BIG 获取": Value Change {
        w311 = u16 1 items=["HPRI"=1, "LPRI"=0] ("priority")
        n116 = event-data() -> ()  [unwired: 1 in, 6 out]
        n117 = property on="Main" class="TabCtl (严格)"("Value"=enum32{"主参数", "模板匹配参数 ", "CCD1 ROI参数", "测试效果"}."测试效果" ("Main")) -> ()  [unwired: 2 in, 2 out]
        n118 = call "Enqueue Element Array.vi"("priority"=w311, "queue index"=0, "error in"=w308, "master data"="ROI BIG 获取", "queue in"=w309) -> ("error out"=w306:errorcluster, "queue out"=w307:T11)  [unwired: 5 in]
      }
      event "测试按钮": Value Change {
        w319 = u16 1 items=["HPRI"=1, "LPRI"=0] ("priority")
        n119 = event-data() -> ()  [unwired: 1 in, 6 out]
        n120 = call "Enqueue Element Array.vi"("priority"=w319, "queue index"=0, "error in"=w316, "master data"="测试按钮", "queue in"=w317) -> ("error out"=w314:errorcluster, "queue out"=w315:T11)  [unwired: 5 in]
        n121 = property on="Main" class="TabCtl (严格)"("Value"=enum32{"主参数", "模板匹配参数 ", "CCD1 ROI参数", "测试效果"}."测试效果" ("Main")) -> ()  [unwired: 2 in, 2 out]
      }
      event "刷新": Value Change {
        n122 = event-data() -> ()  [unwired: 1 in, 6 out]
        n123 = disable-structure shown="禁用" {
          disable-tunnel: w325 -> [w329 _]
          disable-tunnel: w324 -> [w328 _]
          disable-tunnel: [w327 _] -> w323
          disable-tunnel: [w326 _] -> w322
          frame Disabled {
            w331 = u16 1 items=["HPRI"=1, "LPRI"=0] ("priority")
            # "刷新"
            n124 = call "Enqueue Element Array.vi"("priority"=w331, "queue index"=0, "error in"=w328, "master data"="刷新", "queue in"=w329) -> ("error out"=w326:errorcluster, "queue out"=w327:T11)  [unwired: 5 in]
          }
          frame Enabled {
          }
        }
        n125 = property on="Main" class="TabCtl (严格)"("Value"=enum32{"主参数", "模板匹配参数 ", "CCD1 ROI参数", "测试效果"}."模板匹配参数 " ("Main")) -> ()  [unwired: 2 in, 2 out]
      }
    }
    n126 = call "GetSystemTime.vi"() -> ("date/time string"=→"system time":string)  [unwired: 7 in]
  }
  n127 = call "Release Queue Array.vi"("error in"=w3, "queue in"=w1) -> ("error out"=w2:errorcluster)  [unwired: 2 in, 3 out]
  n128 = call "Release Queue Array.vi"("error in"=w6, "queue in"=w1) -> ("error out"=w9:errorcluster)  [unwired: 2 in, 3 out]
  n129 = call "MergeErrors.vi"("error in 3 (no error)"=w2, "error in 4 (no error)"=w9) -> ("error out"=w8:errorcluster)  [unwired: 6 in]
  n130 = call "ExitAppMode.vi"("error in (no error)"=w8) -> ("error out"=w7:errorcluster)  [unwired: 10 in]
  n131 = call <vilib>:"Clear Errors.vi"("error in (no error)"=w7) -> ()  [unwired: 5 in, 2 out]
